vi "UHR-Fleezers Control (host) - Lorentz v2.vi"() -> ()   [LabVIEW 2014] (continued)
                  n2956 = local read "APD 2 Rate (Hz)"() -> (w4355:dbl)
                  n2957 = Multiply(x="Cy5 Fl.  Thresh. (kHz)", y=1000.0) -> (x*y=w4358:dbl)
                  n2958 = Greater?(x=w4355, y=w4358) -> (0:w4354:bool)
                  n2959 = And(x=w4354, y=w4351) -> (x .and. y?=w4352:bool)
                  n2960 = case shown="True" w4352 {
                    frame False {
                    }
                    frame True {
                      n2961 = property on="Green Laser ON" class="Bool (strict)"("Val(Sgnl)"=TRUE ("Value (Signaling)")) -> ()  [unwired: 2 in, 2 out]
                    }
                  }
                  n2962 = node-c288() -> ()  [unwired: 1 in, 1 out]
                }
                n2963 = node-c288(w4349) -> ()  [unwired: 1 out]
              }
              frame #4 {
                w4365 = FALSE ("Value (Signaling)")
                # "lower spot"
                n2964 = local read "Saved Stage Positions"() -> (w4369:dbl[][])
                n2965 = property on="Red Laser ON" class="Bool (strict)"("Val(Sgnl)"=w4365) -> ()  [unwired: 2 in, 2 out]
                n2966 = property on="Green Laser ON" class="Bool (strict)"("Val(Sgnl)"=w4365) -> ()  [unwired: 2 in, 2 out]
                n2967 = local write "Stage Moving"(TRUE ("Stage Moving")) -> ()
                n2968 = local write "Stop assembly line"(FALSE ("Stop assembly line")) -> ()
                n2969 = call "move to saved stage position.vi"("Stage VISA resource name in"=w4366, "Position"=3, "Saved Stage Positions"=w4369) -> ("error out"=w4368:errorcluster)  [unwired: 1 in, 1 out]
                n2970 = local write "Stage Control Serial Error"(w4368) -> ()
              }
              frame #5 {
                w4371 = FALSE ("Stage Moving")
                n2971 = local write "Stage Moving"(w4371) -> ()
                n2972 = local write "AL Running"(w4371) -> ()
                n2973 = call <vilib>:"Beep.vi"() -> ()  [unwired: 3 in, 9 out]
              }
            }
          }
        }
      }
      event "Stop All": Value Change {
        n2974 = event-data() -> ()  [unwired: 7 out]
        n2975 = local read "Stop All"() -> (w4372:bool)
      }
    }
    n2976 = node-c288() -> ()  [unwired: 2 out]
  }
  n2977 = node-c288(i64 1 ("Period"), 1 ("Processor")) -> (w68:T35)  [unwired: 2 in, 2 out]
  n2978 = node-c288(w29) -> ()  [unwired: 1 out]
  n2979 = node-c288(w61) -> ()  [unwired: 1 out]
  n2980 = node-c288(w63) -> ()  [unwired: 1 out]
  n2981 = node-c288(w51) -> ()  [unwired: 1 out]
  n2982 = property on="Saved trap pos" class="WFGraph (strict)"("Visible"=FALSE) -> ()  [unwired: 2 in, 2 out]
  n2983 = property on="Trap Delta Graph" class="WFGraph (strict)"("Visible"=TRUE) -> ()  [unwired: 2 in, 2 out]
  n2984 = disable-structure shown="Disabled" {
    disable-tunnel: w54 -> [w4374 _]
    disable-tunnel: w53 -> [w4373 _]
    frame Disabled {
      n2985 = VISA Close(VISA resource name=w4374, error in (no error)=w4373) -> (error out=w4375:errorcluster)
      n2986 = call <vilib>:"Simple Error Handler.vi"("error in (no error)"=w4375) -> ()  [unwired: 1 in, 8 out]
    }
    frame Enabled {
    }
  }
  n2987 = disable-structure shown="Disabled" {
    disable-tunnel: [w4383 _] -> w15
    disable-tunnel: [w4379 _] -> w14
    disable-tunnel: [w4378 _] -> w13
    disable-tunnel: [w4377 _] -> w12
    disable-tunnel: [w4376 _] -> w11
    frame Disabled {
      # "n samples needed for data"
      n2988 = Unbundle By Name("sound format") -> ("sample rate (S/s)"=w4379:dbl)
      n2989 = call <vilib>:"Sound Output Configure.vi"("number of samples/ch"="number of samples/ch", "sample mode"="sample mode", "sound format"="sound format", "device ID"="device ID") -> ("task ID"=w4383:T50)  [unwired: 6 in, 1 out]
      n2990 = local read "DMA Update Period (s)"() -> (w4380:dbl)
      n2991 = Multiply(x=w4380, y=w4379) -> (x*y=w4378:dbl)
      n2992 = for "Sound time base" {
        N: w4378 -> [_]
        tunnel: [w4387] -> w4381 mode=indexing
        i -> [w4387]
      }
      n2993 = Reciprocal(x=w4379) -> (1/x=w4377:dbl)
      n2994 = Multiply(x=w4381, y=w4377) -> (x*y=w4376:dbl[])
    }
    frame Enabled {
    }
  }
  n2995 = timed-loop "Main data acquisition loop (get data, process data for display, and save data to disk)" {
    tunnel: w10 -> [w4738]
    tunnel: w23 -> [w4737]
    tunnel: [w4765] -> w75
    tunnel: [w4760] -> w74
    timing: w68 -> [_]
    timing-out: [_] -> w67
    tunnel: w45 -> [w4627]
    tunnel: [w4459] -> w16
    tunnel: w15 -> [w4458]
    tunnel: w14 -> [w4456]
    tunnel: w13 -> [w4455]
    tunnel: w12 -> [w4454]
    tunnel: w11 -> [w4453]
    stop <- "Stop All" stop-if-true
    w4403 = 6.0  # clock mult.
    w4402 = 49152000.0  # TCXO frequ.
    w4544 = "Initialize"
    # "Added by Ronen - the limits imposed on amplitudes sent to AOM\nare not explicitly imposed when using intensity feedback. At amplitude of \n~48% FB intensity is ~1.8, if while feedback is on the value passes 1.8, feedback\nis turned off (indication that feedback algorithm overshoots)."
    # "Confocal image scanning disable by Ronen"
    # "List of channels in order (X or Y only):\nT1 X (mV)\nT2 X (mV)\nT1 X (nm)\nT2 X (nm)\nT1 FX (pN)\nT2 FX (pN)\nPosition Difference (nm)\nAPD1\nAPD2\nAPD3"
    # "T2 sum"
    # "T1 sum"
    # "Fluorescence data into FIFO for external control vi's\n(e.g., fluorescence triggering) - Duncan Nall"
    n2996 = node-c288() -> ()  [unwired: 2 out]
    n2997 = First Call?() -> (First Call?: T/F=w4579:bool)
    n2998 = Or(x="Reset", y=w4579) -> (x .or. y?=w4580:bool)
    n2999 = local read "Flushing P1"() -> (w4504:bool)
    n3000 = case "Reset data stream (manual reset or at begining of some rastering and imaging)" shown="True" w4580 {
      tunnel: w4738 -> [w5877 w5885]
      tunnel: w4737 -> [w5876 w5884]
      tunnel: [w5877 w5879] -> w4432
      tunnel: [w5876 w5878] -> w4433
      frame False {
      }
      frame True {
        w5882 = TRUE ("AI to FIFO")
        n3001 = local write "Overflow (data lost)"(FALSE ("Overflow (data lost)")) -> ()
        n3002 = call "reset FPGA DMA.vi"("error in"=w5884, "FPGA VI Reference In"=w5885) -> ("error out"=w5880:errorcluster, "FPGA VI Reference Out"=w5881:T31)
        n3003 = xnode "Read/Write Control"("FPGA VI Reference In"=w5881, "error in"=w5880, "AI to FIFO"=w5882, "APD to FIFO"=w5882) -> ("FPGA VI Reference Out"=w5879:T31, "error out"=w5878:errorcluster)
      }
    }
    n3004 = case shown="False" w4504 {
      frame False {
      }
      frame True {
        n3005 = local read "Flush rate (uL/m) P1"() -> (w4912:dbl)
        n3006 = local read "HP1 Flush Time (s)"() -> (w4921:dbl)
        n3007 = local read "DMA Update Period (s)"() -> (w4915:dbl)
        n3008 = Divide(x=w4912, y=60.0) -> (x/y=w4913:dbl)
        n3009 = Divide(x=w4921, y=w4915) -> (x/y=w4910:dbl)
        n3010 = feedback #4(0) -> (w4919:i32)
        n3011 = Increment(x=w4919) -> (x+1=w4909:i32)
        n3012 = Greater?(x=w4909, y=w4910) -> (0:w4918:bool)
        n3013 = Compound Arithmetic op=MULTIPLY(w4915, w4909, w4913) -> (→"P1 Flush Volume (uL)":dbl)
        n3014 = Divide(x=w4909, y=w4910) -> (x/y=→"P1 Flushing Bar":dbl)
        n3015 = case shown="True" w4918 {
          tunnel: w4909 -> [w4922 _]
          tunnel: [w4922 0] -> w4917
          frame False {
          }
          frame True {
            w4923 = FALSE ("Flushing P1")
            n3016 = local write "Inject Pump 1"(w4923) -> ()
            n3017 = local write "Flushing P1"(w4923) -> ()
            n3018 = property on="Clear Volume P1" class="Bool (strict)"("Val(Sgnl)"=TRUE ("Value (Signaling)")) -> ()  [unwired: 2 in, 2 out]
          }
        }
        n3019 = feedback-in #4(w4917) -> ()
      }
    }
    n3020 = Or(x="Start AOD Scan", y="Trap Raster Scan") -> (x .or. y?=w4700:bool)
    n3021 = case "Start active calibration (oscillate traps precisely)" shown="True" "Active Cal" {
      tunnel: w4433 -> [w4826 w4834]
      tunnel: w4432 -> [w4825 w4835]
      tunnel: [w4826 w4831] -> w4431
      tunnel: [w4825 w4832] -> w4430
      frame False {
      }
      frame True {
        w4827 = TRUE ("APD to FIFO")
        n3022 = call "reset FPGA DMA.vi"("error in"=w4834, "FPGA VI Reference In"=w4835) -> ("error out"=w4828:errorcluster, "FPGA VI Reference Out"=w4829:T31)
        n3023 = local write "Active Cal"(FALSE ("Active Cal")) -> ()
        n3024 = local write "Save Calibration"(TRUE ("Save Calibration")) -> ()
        n3025 = xnode "Read/Write Control"("FPGA VI Reference In"=w4829, "error in"=w4828, "AI to FIFO"=w4827, "APD to FIFO"=w4827) -> ("FPGA VI Reference Out"=w4832:T31, "error out"=w4831:errorcluster)
      }
    }
    n3026 = case "Start AOM raster scan" shown="True" w4700 {
      tunnel: w4430 -> [w5727 w5737]
      tunnel: w4431 -> [w5726 w5736]
      tunnel: [w5727 w5730] -> w4733
      tunnel: [w5726 w5729] -> w4732
      frame False {
      }
      frame True {
        n3027 = case shown="True" "Restart DMA? (AOD)" {
          tunnel: [w5775 w5777] -> w5731
          tunnel: [w5774 w5776] -> w5732
          tunnel: w5737 -> [w5775 w5779]
          tunnel: w5736 -> [w5774 w5778]
          frame False {
          }
          frame True {
            n3028 = local write "Overflow (data lost)"(FALSE ("Overflow (data lost)")) -> ()
            n3029 = call "reset FPGA DMA.vi"("error in"=w5778, "FPGA VI Reference In"=w5779) -> ("error out"=w5776:errorcluster, "FPGA VI Reference Out"=w5777:T31)
          }
        }
        n3030 = local write "Trap Raster Scan"(FALSE ("Trap Raster Scan")) -> ()
        n3031 = case shown="True" "Move MCL Also?" {
          tunnel: w5732 -> [w5740 w5769]
          tunnel: w5731 -> [w5741 w5770]
          tunnel: [w5739 w5773] -> w5730
          tunnel: [w5738 w5772] -> w5729
          frame False {
            w5742 = TRUE ("AI to FIFO")
            n3032 = xnode "Read/Write Control"("FPGA VI Reference In"=w5741, "error in"=w5740, "AI to FIFO"=w5742, "APD to FIFO"=w5742, "Start scan"=w5742) -> ("FPGA VI Reference Out"=w5739:T31, "error out"=w5738:errorcluster)
          }
          frame True {
            w5766 = FALSE ("1D or 2D Scan?")
            w5771 = TRUE ("AI to FIFO")
            # "Count for MCL loop"
            # "N total cycles"
            # "N steps"
            # "V_int"
            n3033 = local read "Scan Range (nm)"() -> (w5748:dbl)
            n3034 = local read "Number of F/B Scans (AOD)"() -> (w5765:u16)
            n3035 = Sign(1:w5748) -> (0:w5747:dbl)
            n3036 = Compound Arithmetic op=MULTIPLY(w5748, "MCL Step Position Ratio", "MCL/AOM Scale Tweak") -> (w5752:dbl)
            n3037 = Negate(x=w5747) -> (-x=w5744:dbl)
            n3038 = Multiply(x=w5744, y="MCL Step Increment (V_int)") -> (x*y=w5746:dbl)
            n3039 = Divide(x=w5752, y="MCL X Cal (nm/V)") -> (x/y=w5758:dbl)
            n3040 = Multiply(x=32767.0 ("y"), y=w5758) -> (x*y=w5764:dbl)
            n3041 = local read "Total Counts (ticks)"() -> (w5749:u16)
            n3042 = local read "Cycles/step (AOD)"() -> (w5760:u64)
            n3043 = local read "Scan steps (AOD)"() -> (w5761:u64)
            n3044 = Divide(x=w5764, y=10.0) -> (x/y=w5757:dbl)
            n3045 = Divide(x=w5757, y="MCL Step Increment (V_int)") -> (x/y=w5755:dbl)
            n3046 = Absolute Value(x=w5755) -> (abs(x)=w5743:dbl)
            n3047 = Compound Arithmetic op=MULTIPLY(w5761, w5760, w5749) -> (w5756:u64)
            n3048 = Divide(x=w5756, y=w5743) -> (x/y=w5753:dbl)
            "MCL Count" <- w5753
            n3049 = xnode "Read/Write Control"("FPGA VI Reference In"=w5770, "error in"=w5769, "Scan steps (MCL)"=w5743, "Number of scans (MCL)"=w5765, "Cycles per step (MCL)"=u64 1, "Scan freq.  increment (MCL)"=w5746, "1D or 2D Scan?"=w5766, "MCL Scan Axis"=w5766, "Cont. Scan (MCL)"=w5766, "MCL count"=w5753) -> ("FPGA VI Reference Out"=w5768:T31, "error out"=w5767:errorcluster)
            n3050 = xnode "Read/Write Control"("FPGA VI Reference In"=w5768, "error in"=w5767, "AI to FIFO"=w5771, "APD to FIFO"=w5771, "Start scan"=w5771, "Start scan (MCL)"=w5771) -> ("FPGA VI Reference Out"=w5773:T31, "error out"=w5772:errorcluster)
            n3051 = local write "MCL Scanning"(w5771) -> ()
            n3052 = local write "wait to reset values"(w5771) -> ()
          }
        }
        "Raster Scanning..." <- TRUE ("Scanning...")
      }
    }
    n3053 = local read "Flushing P3"() -> (w4505:bool)
    n3054 = case "Keep track of when Harvard Pump 3 is done flushing" shown="True" w4505 {
      frame False {
      }
      frame True {
        n3055 = local read "Flush rate (uL/m) P3"() -> (w4929:dbl)
        n3056 = local read "DMA Update Period (s)"() -> (w4931:dbl)
        n3057 = local read "HP3 Flush Time (s)"() -> (w4938:dbl)
        n3058 = Divide(x=w4929, y=60.0) -> (x/y=w4927:dbl)
        n3059 = feedback #5(0) -> (w4936:i32)
        n3060 = Increment(x=w4936) -> (x+1=w4930:i32)
        n3061 = Divide(x=w4938, y=w4931) -> (x/y=w4932:dbl)
        n3062 = Greater?(x=w4930, y=w4932) -> (0:w4935:bool)
        n3063 = Compound Arithmetic op=MULTIPLY(w4931, w4930, w4927) -> (→"P3 Flush Volume (uL)":dbl)
        n3064 = case shown="True" w4935 {
          tunnel: w4930 -> [w4939 _]
          tunnel: [w4939 0] -> w4934
          frame False {
          }
          frame True {
            w4940 = FALSE ("Flushing P3")
            n3065 = local write "Inject Pump 3"(w4940) -> ()
            n3066 = local write "Flushing P3"(w4940) -> ()
            n3067 = property on="Clear Volume P3" class="Bool (strict)"("Val(Sgnl)"=TRUE ("Value (Signaling)")) -> ()  [unwired: 2 in, 2 out]
          }
        }
        n3068 = feedback-in #5(w4934) -> ()
        n3069 = Divide(x=w4930, y=w4932) -> (x/y=→"P3 Flushing Bar":dbl)
      }
    }
    n3070 = And(x="Save scans", y=w4700) -> (x .and. y?=w4731:bool)
    n3071 = Compound Arithmetic op=OR("Start MCL Scan", "Confocal Image", "Confocal Linescan") -> (w4698:bool)
    n3072 = And(x="Save Data (MCL)", y=w4698) -> (x .and. y?=w4730:bool)
    n3073 = case "Start MCL raster scan" shown="True" w4698 {
      tunnel: w4733 -> [w5339 w5355]
      tunnel: w4732 -> [w5338 w5354]
      tunnel: [w5339 w5350] -> w4626
      tunnel: [w5338 w5349] -> w4625
      tunnel: [FALSE w5348] -> w4716
      tunnel: "Start MCL Scan" -> [_ w5343]
      tunnel: "Confocal Image" -> [_ w5342]
      tunnel: "Confocal Linescan" -> [_ _]
      frame False {
      }
      frame True {
        w5348 = TRUE
        n3074 = case shown="True" "Restart DMA? (MCL)" {
          tunnel: [w5400 w5402] -> w5353
          tunnel: [w5399 w5401] -> w5352
          tunnel: w5355 -> [w5400 w5405]
          tunnel: w5354 -> [w5399 w5404]
          frame False {
          }
          frame True {
            n3075 = call "reset FPGA DMA.vi"("error in"=w5404, "FPGA VI Reference In"=w5405) -> ("error out"=w5401:errorcluster, "FPGA VI Reference Out"=w5402:T31)
            n3076 = local write "Overflow (data lost)"(FALSE ("Overflow (data lost)")) -> ()
          }
        }
        n3077 = case shown="False" w5343 {
          selector: w5343 -> [_ w5359]
          tunnel: w5342 -> [w5358 _]
          tunnel: [w5358 w5359] -> w5341
          frame False {
            n3078 = property on="2D or 1D Scan" class="Bool (strict)"("Val(Sgnl)"=w5358) -> ()  [unwired: 2 in, 2 out]
            n3079 = property on="Confocal Image" class="Bool (strict)"("Value"=FALSE ("Start Confocal Map")) -> ()  [unwired: 2 in, 2 out]
          }
          frame True {
          }
        }
        n3080 = local write "MCL Scanning"(w5348) -> ()
        n3081 = local read "AO1"() -> (w5345:dbl)
        n3082 = local read "AO2"() -> (w5344:dbl)
        n3083 = case shown="True" "Center Scan" {
          tunnel: w5353 -> [w5366 w5398]
          tunnel: w5352 -> [w5365 w5397]
          tunnel: [w5364 w5396] -> w5350
          tunnel: [w5363 w5395] -> w5349
          tunnel: [w5361 w5382] -> w5347
          tunnel: [w5360 w5381] -> w5346
          tunnel: w5345 -> [w5361 w5387]
          tunnel: w5344 -> [w5360 w5390]
          tunnel: w5341 -> [_ _]
          frame False {
            w5362 = TRUE ("AI to FIFO")
            n3084 = xnode "Read/Write Control"("FPGA VI Reference In"=w5366, "error in"=w5365, "AI to FIFO"=w5362, "APD to FIFO"=w5362, "Start scan (MCL)"=w5362) -> ("FPGA VI Reference Out"=w5364:T31, "error out"=w5363:errorcluster)
          }
          frame True {
            w5394 = TRUE ("AI to FIFO")
            n3085 = local read "Scan steps (MCL)"() -> (w5373:u64)
            n3086 = local read "Scan lines (y)"() -> (w5369:u64)
            n3087 = local read "Fast Scan Dir"() -> (w5380:bool)
            n3088 = local read "Actual MCL Inc (V)"() -> (w5370:dbl)
            n3089 = Decrement(x=w5369) -> (x-1=w5368:u64)
            n3090 = Decrement(x=w5373) -> (x-1=w5372:u64)
            n3091 = Multiply(x=w5370, y=w5368) -> (x*y=w5367:dbl)
            n3092 = Divide(x=w5367, y=2.0) -> (x/y=w5377:dbl)
            n3093 = Multiply(x=w5370, y=w5372) -> (x*y=w5371:dbl)
            n3094 = Divide(x=w5371, y=2.0) -> (x/y=w5376:dbl)
            n3095 = Select(t=w5376, s=w5380, f=w5377) -> (s? t:f=w5375:dbl)
            n3096 = Select(t=w5377, s=w5380, f=w5376) -> (s? t:f=w5379:dbl)
            n3097 = Subtract(x=w5387, y=w5379) -> (x-y=w5378:dbl)
            n3098 = Subtract(x=w5390, y=w5375) -> (x-y=w5374:dbl)
            n3099 = local read "2D or 1D Scan"() -> (w5392:bool)
            n3100 = Not(x=w5380) -> (.not. x?=w5386:bool)
            n3101 = Not(x=w5392) -> (.not. x?=w5388:bool)
            n3102 = And(x=w5380, y=w5388) -> (x .and. y?=w5389:bool)
            n3103 = And(x=w5388, y=w5386) -> (x .and. y?=w5391:bool)
            n3104 = Select(t=w5390, s=w5391, f=w5374) -> (s? t:f=w5381:dbl)
            n3105 = Select(t=w5387, s=w5389, f=w5378) -> (s? t:f=w5382:dbl)
            n3106 = call "Volt to I16.vi"("Voltage In"=w5382) -> ("I16 Voltage Out"=w5385:i16)
            n3107 = call "Volt to I16.vi"("Voltage In"=w5381) -> ("I16 Voltage Out"=w5384:i16)
            n3108 = xnode "Read/Write Control"("FPGA VI Reference In"=w5398, "error in"=w5397, "AI to FIFO"=w5394, "APD to FIFO"=w5394, "Start scan (MCL)"=w5394, "AO1"=w5385, "AO2"=w5384) -> ("FPGA VI Reference Out"=w5396:T31, "error out"=w5395:errorcluster)
          }
        }
        "Initial Y" <- w5347
        "Initial X" <- w5346
        n3109 = local write "Tab Control 6"(T3."Imaging" ("Tab Control 6")) -> ()
        "wait to reset values" <- w5348
      }
    }
    n3110 = local read "APD Elements/DMA read"() -> (w4475:u32)
    n3111 = local read "Trap AI Elements/DMA read"() -> (w4679:u32)
    n3112 = xnode "Get APD Data"("FPGA VI Reference In"=w4626, "error in"=w4625, "Number of Elements"=w4475, "Timeout (ms)"=-1) -> ("Data"=w4654:void[], "Elements Remaining"=→"APD FIFO Elements Remaining")  [unwired: 2 out]
    n3113 = local read "Trap Pos Elements/DMA read"() -> (w4622:u32)
    n3114 = xnode "Invoke Method"("FPGA VI Reference In"=w4626, "error in"=w4625, "Number of Elements"=w4622, "Timeout (ms)"=-1) -> ("Data"=w4586:void[], "Elements Remaining"=→"Trap Pos FIFO El Remaining")  [unwired: 2 out]
    n3115 = xnode "Get Trap Data"("FPGA VI Reference In"=w4626, "error in"=w4625, "Number of Elements"=w4679, "Timeout (ms)"=-1 ("Timeout")) -> ("FPGA VI Reference Out"=w4401:T31, "error out"=w4522:errorcluster, "Data"=w4587:void[], "Elements Remaining"=w4773)
    "FIFO El. Rem." <- w4773
    n3116 = local read "DMA Update Period (s)"() -> (w4680:dbl)
    n3117 = local read "Trap AI FIFO Depth"() -> (w4775:u32)
    n3118 = local read "Number of APDs"() -> (w4494:u8)
    n3119 = Decimate 1D Array(w4586) -> (w4583:void[], w4585:void[], w4584:void[])
    n3120 = feedback #6(0.0) -> (w4615:dbl)
    n3121 = Add(x=w4680, y=w4615) -> (x+y=w4750:dbl)
    n3122 = feedback-in #6(w4750) -> ()
    n3123 = To Time Stamp(1:w4615) -> (0:w4614:timestamp)
    n3124 = Subtract(x=w4775, y=w4679) -> (x-y=w4774:u32)
    n3125 = To Unsigned Long Integer(number=w4583) -> (unsigned 32bit integer=w4582:u32[])
    n3126 = Join Numbers(hi=w4585, lo=w4584) -> ((hi.lo)=w4581:u32)
    n3127 = Divide(x=w4773, y=w4774) -> (x/y=w4772:dbl)
    "Buffer Status" <- w4772
    n3128 = case "Deinterlace APD signals" shown="3, Default" w4494 {
      tunnel: [w4902 w4908] -> w4474
      tunnel: w4654 -> [w4903 w4907]
      tunnel: [w4901 w4906] -> w4473
      tunnel: [w4900 w4904] -> w4422
      frame 3, Default {
        n3129 = Decimate 1D Array "APD signals"(w4903) -> (w4902:void[], w4901:void[], w4900:void[])
      }
      frame 2 {
        n3130 = Decimate 1D Array "APD signals"(w4907) -> (w4908:void[], w4906:void[])
        n3131 = Multiply(x=w4906, y=u32 0) -> (x*y=w4904:u32)
      }
    }
    n3132 = Join Numbers(hi=w4582, lo=w4581) -> ((hi.lo)=w4575:u64[])
    n3133 = call "IR AOM word to freq - vec.vi"("Frequency Word In (double vec)"=w4575) -> ("Frequency Out"=w4621:dbl[])
    n3134 = Equal?(x=w4772, y=1.0) -> (x = y?=w4770:bool)
    n3135 = case "Alert buffer overflow" shown="False" w4770 {
      frame False {
      }
      frame True {
        n3136 = call <vilib>:"Beep.vi"() -> ()  [unwired: 3 in, 9 out]
        "Overflow (data lost)" <- TRUE ("Overflow (data lost)")
      }
    }
    n3137 = Decimate 1D Array(w4621) -> (w4620:dbl[], w4619:dbl[])
    n3138 = Build Array(w4620, w4619) -> (w4618:dbl[][])
    n3139 = Bundle(w4474, w4473, w4422) -> (w4478:cluster{void[], void[], u32})  [unwired: 1 in]
    n3140 = Build Array(w4474, w4473, w4422) -> (w4713:u32[])
    n3141 = for {
      tunnel: w4474 -> [w4898] mode=indexing
      n3142 = call "Smart Buffer (DBL) 1.vi"("new element [write]"=w4898, "mode"=T33."write") -> ()  [unwired: 4 in, 6 out]
    }
    n3143 = local read "APD Integration Time (s)"() -> (w4489:dbl)
    n3144 = To Double Precision Float(number=w4713) -> (double precision float=w4714:dbl[])
    n3145 = feedback #7 "APD3"(w4422) -> (w4423:u32)
    n3146 = feedback #8 "APD2"(w4473) -> (w4644:void[])
    n3147 = feedback #9 "APD1"(w4474) -> (w4712:void[])
    n3148 = Build Array(w4423, w4422) -> (w4421:u32[])
    n3149 = Build Array (concatenate)(w4644, w4473) -> (w4643:void[])
    n3150 = Build Array (concatenate)(w4712, w4474) -> (w4709:void[])
    n3151 = for {
      tunnel: w4473 -> [w4897] mode=indexing
      n3152 = call "Smart Buffer (DBL) 2.vi"("new element [write]"=w4897, "mode"=T33."write") -> ()  [unwired: 4 in, 6 out]
    }
    n3153 = Array Size(array=w4709) -> (size(s)=w4706:i32)
    n3154 = Array Size(array=w4474) -> (size(s)=w4708:i32)
    n3155 = Multiply(x=w4708, y="APD Ave N") -> (x*y=w4707:dbl)
    n3156 = Greater?(x=w4706, y=w4707) -> (0:w4710:bool)
    n3157 = Bundle("APD 1", "APD 2", "APD 3") -> (w4744:cluster{string, string, string})  [unwired: 1 out]
    n3158 = local read "Trap Sets"() -> (w4678:u32)
    n3159 = case shown="True" w4710 {
      tunnel: w4709 -> [w5154 w5163]
      tunnel: [w5154 w5161] -> w4685
      tunnel: w4707 -> [_ w5156]
      tunnel: w4706 -> [_ w5162]
      tunnel: w4643 -> [w5153 w5160]
      tunnel: [w5153 w5159] -> w4641
      tunnel: w4421 -> [w5152 w5158]
      tunnel: [w5152 w5155] -> w4490
      frame False {
      }
      frame True {
        n3160 = Subtract(x=w5162, y=w5156) -> (x-y=w5157:dbl)
        n3161 = Array Subset "APD3"(array=w5158, index=w5157, length=w5156) -> (w5155:u32[])
        n3162 = Array Subset "APD2"(array=w5160, index=w5157, length=w5156) -> (w5159:void[])
        n3163 = Array Subset "APD1"(array=w5163, index=w5157, length=w5156) -> (w5161:void[])
      }
    }
    n3164 = feedback-in #7(w4490) -> ()
    n3165 = feedback-in #8(w4641) -> ()
    n3166 = feedback-in #9(w4685) -> ()
    n3167 = Cluster To Array(cluster=w4744) -> (array=w4741:string[])
    n3168 = for "APD" {
      tunnel: w4714 -> [w5410] mode=indexing
      tunnel: w4489 -> [w5417]
      tunnel: [w5413] -> w4645 mode=indexing
      tunnel: "APD Disp. Scale" -> [w5414]
      tunnel: w4741 -> [w5412] mode=indexing
      tunnel: "APD Disp. Downsample" -> [w5408]
      tunnel: [w5411] -> w4740
      workers-P: _ -> [_]
      tunnel: w4614 -> [w5407]
      n3169 = call "integrate 1D array interval - double.vi"("Ave N"=w5408, "Array In"=w5410) -> ("Array Out"=w5409:dbl[])  [unwired: 1 out]
      n3170 = Multiply(x=w5417, y=w5408) -> (x*y=w5411:dbl)
      n3171 = Divide(x=w5409, y=w5414) -> (x/y=w5415:dbl[])
      n3172 = Bundle By Name("t0"=w5407, "Y"=w5415, "dt"=w5411) -> (w5416:waveform(dbl))  [unwired: 1 out]
      n3173 = Set Waveform Attribute(5:w5412, 6:"NI_ChannelName" ("name"), 7:w5416) -> (3:w5413:waveform(dbl))  [unwired: 1 in, 2 out]
    }
    "APD Display Period (s)" <- w4740
    n3174 = Reciprocal(x=w4740) -> (1/x=→"APD Display Freq. (Hz)":dbl)
    n3175 = case "Deinterlace trap data, average down PSD" shown="2" w4678 {
      tunnel: w4587 -> [w5435 w5500]
      tunnel: [w5432 w5497] -> w4673
      tunnel: [w5435 w5499] -> w4578
      tunnel: "Detector Type" -> [w5434 w5495]
      tunnel: [w5433 w5498] -> w4672
      tunnel: [w5431 w5496] -> w4748
      frame 1, Default {
        n3176 = Divide(x=w5435, y=3276.7) -> (x/y=w5436:dbl)
        n3177 = Decimate 1D Array(w5436) -> (w5445:dbl[], w5444:dbl[], w5443:dbl[], w5442:dbl[], w5441:dbl[], w5440:dbl[], w5439:dbl[], w5438:dbl[])
        n3178 = case shown="\"IR-QPD + PSD + FB-QPD position\"" w5434 {
          tunnel: w5445 -> [w5469 w5494]
          tunnel: w5444 -> [w5468 w5493]
          tunnel: w5443 -> [w5453 w5471]
          tunnel: w5442 -> [w5454 w5481]
          tunnel: w5441 -> [w5467 w5492]
          tunnel: w5440 -> [w5466 w5491]
          tunnel: w5439 -> [w5450 w5472]
          tunnel: w5438 -> [w5449 w5470]
          tunnel: [w5448 w5478] -> w5433
          tunnel: [w5447 w5477] -> w5432
          tunnel: [w5446 w5476] -> w5431
          frame "IR-QPD + PSD + FB-QPD", Default {
            w5446 = 0  # Channel pattern
            n3179 = Divide(x=w5469, y=w5454) -> (x/y=w5456:dbl[])
            n3180 = Divide(x=w5468, y=w5454) -> (x/y=w5455:dbl[])
            n3181 = Divide(x=w5467, y=w5450) -> (x/y=w5452:dbl[])
            n3182 = Divide(x=w5466, y=w5449) -> (x/y=w5451:dbl[])
            n3183 = Build Array(w5456, w5455, w5454, w5453, w5452, w5451, w5450, w5449) -> (w5447:dbl[][])
            n3184 = Bundle("T1 Y", "T1 X", "T1 Sum", "FB Sum", "PSD Y", "PSD X", "PSD Y Sum", "PSD X Sum") -> (w5465:T57)  [unwired: 1 out]
            n3185 = Cluster To Array(cluster=w5465) -> (array=w5448:string[])
          }
          frame "IR-QPD + PSD + FB-QPD position" {
            w5476 = 3  # Channel pattern
            n3186 = Negate(x=w5472) -> (-x=w5473:dbl[])
            n3187 = Divide(x=w5494, y=w5481) -> (x/y=w5483:dbl[])
            n3188 = Divide(x=w5493, y=w5481) -> (x/y=w5482:dbl[])
            n3189 = Divide(x=w5492, y=w5472) -> (x/y=w5480:dbl[])
            n3190 = Divide(x=w5491, y=w5473) -> (x/y=w5479:dbl[])
            n3191 = Build Array(w5483, w5482, w5481, w5470, w5471, w5480, w5479, w5472) -> (w5477:dbl[][])
            n3192 = Bundle("T1 Y", "T1 X", "T1 Sum", "FB X", "FB Sum", "PSD Y", "PSD X", "PSD Y Sum") -> (w5490:T57)  [unwired: 1 out]
            n3193 = Cluster To Array(cluster=w5490) -> (array=w5478:string[])
          }
        }
      }
      frame 2 {
        n3194 = case shown="\"IR-QPD + PSD + FB-QPD X position\", Default" w5495 {
          tunnel: w5500 -> [w5562 w5634 w5705]
          tunnel: [w5501 w5625 w5636] -> w5499
          tunnel: [w5528 w5616 w5683] -> w5498
          tunnel: [w5527 w5579 w5650] -> w5497
          tunnel: [w5521 w5614 w5681] -> w5496
          frame "IR-QPD + PSD + FB-QPD" {
            w5521 = 1  # Channel pattern
            # "time average x2 the 4th signal and the 4 psd signals (detection laser)"
            # "deinterlace 3 signals from qpd"
            n3195 = Decimate 1D Array(w5562) -> (w5561:void[], w5560:void[], w5526:void[], w5559:void[], w5549:void[], w5547:void[], w5546:void[], w5544:void[])
            n3196 = Decimate 1D Array(w5526) -> (w5525:void[], w5524:void[])
            n3197 = Decimate 1D Array(w5561) -> (w5558:void[], w5530:void[])
            n3198 = Decimate 1D Array(w5560) -> (w5557:void[], w5555:void[])
            n3199 = Decimate 1D Array(w5559) -> (w5556:void[], w5554:void[])
            n3200 = call "downsample 1D array - double.vi"("Ave N"=2.0, "Array In"=w5549) -> ("Array Out"=w5548:dbl[])  [unwired: 1 out]
            n3201 = call "downsample 1D array - double.vi"("Ave N"=2.0, "Array In"=w5547) -> ("Array Out"=w5529:dbl[])  [unwired: 1 out]
            n3202 = call "downsample 1D array - double.vi"("Ave N"=2.0, "Array In"=w5546) -> ("Array Out"=w5545:dbl[])  [unwired: 1 out]
            n3203 = call "downsample 1D array - double.vi"("Ave N"=2.0, "Array In"=w5544) -> ("Array Out"=w5543:dbl[])  [unwired: 1 out]
            n3204 = Interleave 1D Arrays(w5558, w5557, w5556, w5530, w5555, w5554, w5525, w5524, w5548, w5529, w5545, w5543) -> (w5542:dbl[])
            n3205 = Divide(x=w5542, y=3276.7) -> (x/y=w5541:dbl[])
            n3206 = Decimate 1D Array(w5541) -> (w5540:dbl[], w5539:dbl[], w5538:dbl[], w5537:dbl[], w5536:dbl[], w5535:dbl[], w5523:dbl[], w5522:dbl[], w5534:dbl[], w5533:dbl[], w5532:dbl[], w5531:dbl[])
            n3207 = Divide(x=w5540, y=w5538) -> (x/y=w5508:dbl[])
            n3208 = Divide(x=w5539, y=w5538) -> (x/y=w5507:dbl[])
            n3209 = Divide(x=w5537, y=w5535) -> (x/y=w5506:dbl[])
            n3210 = Divide(x=w5536, y=w5535) -> (x/y=w5505:dbl[])
            n3211 = Divide(x=w5534, y=w5532) -> (x/y=w5504:dbl[])
            n3212 = Divide(x=w5533, y=w5531) -> (x/y=w5503:dbl[])
            n3213 = Build Array(w5508, w5507, w5538, w5506, w5505, w5535, w5523, w5522, w5504, w5503, w5532, w5531) -> (w5527:dbl[][])
            n3214 = Bundle("T1 Y", "T1 X", "T1 Sum", "T2 Y", "T2 X", "T2 Sum", "T1 FB Sum", "T2 FB Sum", "PSD Y", "PSD X", "PSD Y Sum", "PSD X Sum") -> (w5509:T58)  [unwired: 1 out]
            n3215 = To Word Integer(number=w5542) -> (16bit integer=w5501:i16[])
            n3216 = Cluster To Array(cluster=w5509) -> (array=w5528:string[])
          }
          frame "IR-QPD + PSD + FB-QPD X position", Default {
            w5614 = 2  # Channel pattern
            # "time average x2 the 3 psd signals (detection laser)"
            # "deinterlace 3 signals from qpds"
            n3217 = Decimate 1D Array(w5634) -> (w5633:void[], w5632:void[], w5615:void[], w5631:void[], w5577:void[], w5574:void[], w5571:void[], w5602:void[])
            n3218 = Select(t=i16 -1, s="Flip X Sign", f=i16 1) -> (s? t:f=w5567:i16)
            n3219 = Multiply(x=w5632, y=w5567) -> (x*y=w5568:i16)
            n3220 = Decimate 1D Array(w5615) -> (w5600:void[], w5598:void[])
            n3221 = Decimate 1D Array(w5633) -> (w5630:void[], w5617:void[])
            n3222 = Decimate 1D Array(w5568) -> (w5629:dbl[], w5627:dbl[])
            n3223 = Decimate 1D Array(w5631) -> (w5628:void[], w5626:void[])
            n3224 = Decimate 1D Array(w5602) -> (w5601:void[], w5599:void[])
            n3225 = call "downsample 1D array - I16.vi"("Ave N"=2.0, "Array In"=w5577) -> ("Array Out"=w5575:i16[])  [unwired: 1 in]
            n3226 = call "downsample 1D array - I16.vi"("Ave N"=2.0, "Array In"=w5571) -> ("Array Out"=w5569:i16[])  [unwired: 1 in]
            n3227 = call "downsample 1D array - I16.vi"("Ave N"=2.0, "Array In"=w5574) -> ("Array Out"=w5572:i16[])  [unwired: 1 in]
            n3228 = Interleave 1D Arrays(w5630, w5629, w5628, w5617, w5627, w5626, w5601, w5600, w5599, w5598, w5575, w5572, w5569) -> (w5625:dbl[])
            n3229 = Divide(x=w5625, y=3276.7) -> (x/y=w5624:dbl[])
            n3230 = Decimate 1D Array(w5624) -> (w5623:dbl[], w5622:dbl[], w5621:dbl[], w5620:dbl[], w5619:dbl[], w5618:dbl[], w5590:dbl[], w5588:dbl[], w5587:dbl[], w5585:dbl[], w5584:dbl[], w5583:dbl[], w5580:dbl[])
            n3231 = Negate(x=w5580) -> (-x=w5578:dbl[])
            n3232 = Divide(x=w5584, y=w5580) -> (x/y=w5582:dbl[])
            n3233 = Divide(x=w5583, y=w5578) -> (x/y=w5581:dbl[])
            n3234 = Divide(x=w5623, y=w5621) -> (x/y=w5606:dbl[])
            n3235 = Divide(x=w5622, y=w5621) -> (x/y=w5605:dbl[])
            n3236 = Divide(x=w5620, y=w5618) -> (x/y=w5604:dbl[])
            n3237 = Divide(x=w5619, y=w5618) -> (x/y=w5603:dbl[])
            n3238 = Divide(x=w5590, y=w5588) -> (x/y=w5589:dbl[])
            n3239 = Divide(x=w5587, y=w5585) -> (x/y=w5586:dbl[])
            n3240 = Build Array(w5606, w5605, w5621, w5604, w5603, w5618, w5589, w5588, w5586, w5585, w5582, w5581, w5580) -> (w5579:dbl[][])
            n3241 = Bundle("T1 Y", "T1 X", "T1 Sum", "T2 Y", "T2 X", "T2 Sum", "T1 FB X", "T1 FB Sum", "T2 FB X", "T2 FB Sum", "PSD Y", "PSD X", "PSD Y Sum") -> (w5607:T59)  [unwired: 1 out]
            n3242 = Cluster To Array(cluster=w5607) -> (array=w5616:string[])
          }
          frame "IR-QPD + PSD + FB-QPD XY positions" {
            w5681 = 4  # Channel pattern
            # "time average x2 the 3 psd signals (detection laser)"
            # "deinterlace 3 signals from qpds"
            n3243 = Decimate 1D Array(w5705) -> (w5704:void[], w5703:void[], w5682:void[], w5702:void[], w5648:void[], w5694:void[], w5693:void[], w5670:void[])
            n3244 = Decimate 1D Array "Feedback Sum"(w5682) -> (w5666:void[], w5664:void[])
            n3245 = Decimate 1D Array "QPD Y"(w5704) -> (w5701:void[], w5684:void[])
            n3246 = Decimate 1D Array "QPD X"(w5703) -> (w5700:void[], w5698:void[])
            n3247 = Decimate 1D Array "Feedback Y"(w5648) -> (w5647:void[], w5646:void[])
            n3248 = Decimate 1D Array "QPD Sum"(w5702) -> (w5699:void[], w5697:void[])
            n3249 = Decimate 1D Array "Feedback X"(w5670) -> (w5667:void[], w5665:void[])
            n3250 = call "downsample 1D array - double.vi"("Ave N"=2.0, "Array In"=w5694) -> ("Array Out"=w5669:dbl[])  [unwired: 1 out]
            n3251 = call "downsample 1D array - double.vi"("Ave N"=2.0, "Array In"=w5693) -> ("Array Out"=w5668:dbl[])  [unwired: 1 out]
            n3252 = Interleave 1D Arrays(w5701, w5700, w5699, w5684, w5698, w5697, w5647, w5667, w5666, w5646, w5665, w5664, w5669, w5668) -> (w5692:dbl[])
            n3253 = Divide(x=w5692, y=3276.7) -> (x/y=w5691:dbl[])
            n3254 = Decimate 1D Array(w5691) -> (w5690:dbl[], w5689:dbl[], w5688:dbl[], w5687:dbl[], w5686:dbl[], w5685:dbl[], w5643:dbl[], w5657:dbl[], w5641:dbl[], w5642:dbl[], w5655:dbl[], w5639:dbl[], w5653:dbl[], w5651:dbl[])
            n3255 = Negate(x=w5651) -> (-x=w5649:dbl[])
            n3256 = Divide(x=w5653, y=w5649) -> (x/y=w5652:dbl[])
            n3257 = Divide(x=w5642, y=w5639) -> (x/y=w5638:dbl[])
            n3258 = Divide(x=w5643, y=w5641) -> (x/y=w5640:dbl[])
            n3259 = Divide(x=w5690, y=w5688) -> (x/y=w5674:dbl[])
            n3260 = Divide(x=w5689, y=w5688) -> (x/y=w5673:dbl[])
            n3261 = Divide(x=w5687, y=w5685) -> (x/y=w5672:dbl[])
            n3262 = Divide(x=w5686, y=w5685) -> (x/y=w5671:dbl[])
            n3263 = Divide(x=w5657, y=w5641) -> (x/y=w5656:dbl[])
            n3264 = Divide(x=w5655, y=w5639) -> (x/y=w5654:dbl[])
            n3265 = Build Array(w5674, w5673, w5688, w5672, w5671, w5685, w5640, w5656, w5641, w5638, w5654, w5639, w5652, w5651) -> (w5650:dbl[][])
            n3266 = Bundle("T1 Y", "T1 X", "T1 Sum", "T2 Y", "T2 X", "T2 Sum", "T1 FB Y", "T1 FB X", "T1 FB Sum", "T2 FB Y", "T2 FB X", "T2 FB Sum", "PSD X", "PSD Y Sum") -> (w5637:T60)  [unwired: 1 out]
            n3267 = To Word Integer(number=w5692) -> (16bit integer=w5636:i16[])
            n3268 = Cluster To Array(cluster=w5637) -> (array=w5683:string[])
          }
        }
      }
    }
    "AI labels" <- w4672
    n3269 = local read "APD Integration Time (s)"() -> (w4650:dbl)
    n3270 = Array Size(array=w4685) -> (size(s)=w4705:i32)
    n3271 = call <vilib>:"Std Deviation and Variance.vi"("X"=w4641) -> ("standard deviation"=w4640:dbl)  [unwired: 1 in, 2 out]
    n3272 = Add Array Elements(numeric array=w4641) -> (sum=w4642:dbl)
    n3273 = Add Array Elements(numeric array=w4685) -> (sum=w4715:dbl)
    n3274 = call <vilib>:"Std Deviation and Variance.vi"("X"=w4685) -> ("standard deviation"=w4684:dbl)  [unwired: 1 in, 2 out]
    n3275 = Divide(x=w4640, y=w4489) -> (x/y=w4637:dbl)
    "Rate sigma (Hz) 2" <- w4637
    n3276 = Multiply(x=w4489, y=w4705) -> (x*y=w4491:dbl)
    "Int. Time (s)" <- w4491
    n3277 = Divide(x=w4642, y=w4491) -> (x/y=w4638:dbl)
    "APD 2 Rate (Hz)" <- w4638
    n3278 = Multiply(x="APD Disp. Scale", y=w4645) -> (x*y=w4652:waveform(dbl)[])
    n3279 = Divide(x=w4715, y=w4491) -> (x/y=w4682:dbl)
    "APD 1 Rate (Hz)" <- w4682
    n3280 = Divide(x=w4684, y=w4489) -> (x/y=w4683:dbl)
    "Rate sigma (Hz)" <- w4683
    n3281 = Divide(x=w4637, y=w4638) -> (x/y=→"Sigma/Mean 2":dbl)
    n3282 = Multiply(x="APD Disp. Downsample", y=w4650) -> (x*y=w4648:dbl)
    n3283 = Divide(x=w4683, y=w4682) -> (x/y=→"Sigma/Mean":dbl)
    n3284 = Divide(x=w4652, y=w4648) -> (x/y=w4481:waveform(dbl)[])
    n3285 = Index Array(array=w4481, index=0) -> (element=w4634:waveform(dbl))
    n3286 = Index Array(array=w4481, index=1) -> (element=w4632:waveform(dbl))
    n3287 = Index Array(array=w4481, index=2) -> (element=w4483:waveform(dbl))
    n3288 = Subtract(x=w4634, y="APD 1 Offset") -> (x-y=w4630:waveform(dbl))
    n3289 = Subtract(x=w4632, y="APD 2 Offset") -> (x-y=w4629:waveform(dbl))
    n3290 = Subtract(x=w4483, y="APD 3 Offset") -> (x-y=w4480:waveform(dbl))
    n3291 = Add Array Elements(numeric array=w4490) -> (sum=w4493:u32)
    n3292 = call <vilib>:"Std Deviation and Variance.vi"("X"=w4490) -> ("standard deviation"=w4492:dbl)  [unwired: 1 in, 2 out]
    n3293 = Build Array(w4630, w4629, w4480) -> (→"APD Chart":waveform(dbl)[])
    n3294 = Divide(x=w4493, y=w4491) -> (x/y=w4487:dbl)
    "APD 3 Rate (Hz)" <- w4487
    n3295 = Divide(x=w4492, y=w4489) -> (x/y=w4488:dbl)
    "Rate sigma (Hz) 3" <- w4488
    n3296 = Divide(x=w4488, y=w4487) -> (x/y=→"Sigma/Mean 3":dbl)
    n3297 = xnode "Read/Write Control"("FPGA VI Reference In"=w4401) -> ("FPGA VI Reference Out"=w4400:T31, "BD1 Frequency Out 1"=w4399:u64)  [unwired: 1 in, 1 out]
    n3298 = local read "Data Period (s)"() -> (w4537:dbl)
    n3299 = local read "BD 1 Frequency 2 (MHz)"() -> (w4570:dbl)
    n3300 = local read "BD 1 Frequency 1 (MHz)"() -> (w4571:dbl)
    n3301 = Decimate 1D Array(w4578) -> (w4602:dbl[], w4601:dbl[], w4599:dbl[], w4598:dbl[])  [unwired: 9 out]
    n3302 = Multiply(x=w4537, y="Trap Pos. Disp. Downsample") -> (x*y=w4535:dbl)
    n3303 = Divide(x=w4602, y=w4601) -> (x/y=w4603:dbl[])
    n3304 = Divide(x=w4599, y=w4598) -> (x/y=w4600:dbl[])
    n3305 = local read "AOM X Cal (nm/MHz)"() -> (w4568:dbl)
    n3306 = Split 1D Array(array=w4603, index="N El. to Ave.") -> (second subarray=w4606:dbl[])  [unwired: 1 out]
    n3307 = Split 1D Array(array=w4600, index="N El. to Ave.") -> (second subarray=w4605:dbl[])  [unwired: 1 out]
    n3308 = Multiply(x=w4537, y="Trap Disp. Downsample") -> (x*y=w4616:dbl)
    "Display Period (s)" <- w4616
    n3309 = for "Trap AI" {
      tunnel: [w5430] -> w4446 mode=indexing
      tunnel: w4614 -> [w5421]
      tunnel: "Trap Disp. Downsample" -> [w5428]
      tunnel: w4673 -> [w5426] mode=indexing
      tunnel: w4537 -> [w5425]
      tunnel: w4672 -> [w5424] mode=indexing
      tunnel: [w5423] -> w4647 mode=indexing
      tunnel: w4616 -> [w5422]
      workers-P: _ -> [_]
      n3310 = Bundle By Name("Y"=w5426, "dt"=w5425) -> (w5427:waveform(dbl))  [unwired: 1 out]
      n3311 = Set Waveform Attribute(5:w5424, 6:"NI_ChannelName" ("name"), 7:w5427) -> (3:w5423:waveform(dbl))  [unwired: 1 in, 2 out]
      n3312 = call "downsample 1D array - double.vi"("Ave N"=w5428, "Array In"=w5426) -> ("Array Out"=w5429:dbl[])  [unwired: 1 out]
      n3313 = Bundle By Name(cluster=w5423, "t0"=w5421, "Y"=w5429, "dt"=w5422) -> (w5430:waveform(dbl))
    }
    n3314 = Bundle("BD 1 Frequency 1 (MHz)"=w4571, "BD 1 Frequency 2 (MHz)"=w4570) -> (w4572:T61)  [unwired: 1 out]
    n3315 = call-poly <vilib>:"Mean.vi"("X"=w4605) -> ("mean"=w4593:dbl)  [unwired: 1 out]
    n3316 = call-poly <vilib>:"Mean.vi"("X"=w4606) -> ("mean"=w4594:dbl)  [unwired: 1 out]
    n3317 = local read "BD 1 Frequency 2 (MHz)"() -> (w4411:dbl)
    n3318 = Reciprocal(x=w4616) -> (1/x=→"Trap Disp. Freq. (Hz)":dbl)
    n3319 = Cluster To Array(cluster=w4572) -> (array=w4569:dbl[])
    n3320 = To Double Precision Float(number=w4399) -> (double precision float=w4404:dbl)
    n3321 = Multiply(x=w4402, y=w4403) -> (x*y=w4405:dbl)
    n3322 = local read "Trap X AI1 (DMA)"() -> (w4604:T16)
    n3323 = Multiply(x=w4404, y=w4405) -> (x*y=w4406:dbl)
    n3324 = local read "Data points/scans (MCL)"() -> (w4725:dbl)
    n3325 = To Fixed-Point(number=w4593) -> (fixed-point=w4591:fxp<+/-,16,1>)  [unwired: 1 in]
    n3326 = To Fixed-Point(number=w4594) -> (fixed-point=w4592:fxp<+/-,16,1>)  [unwired: 1 in]
    n3327 = Scale By Power Of 2(n=-48, x=w4406) -> (x*2^n=w4408:dbl)
    n3328 = Bundle("Trap 1 Pos.", "Trap 2 Pos.") -> (w4613:cluster{string, string})  [unwired: 1 out]
    n3329 = Divide(x=w4408, y=1000000.0) -> (x/y=w4410:dbl)
    n3330 = Bundle By Name(cluster=w4604, "Set 1"=w4592, "Set 2"=w4591) -> (→"Trap X AI1 (DMA)":T16)
    n3331 = Cluster To Array(cluster=w4613) -> (array=w4610:string[])
    n3332 = Subtract(x=w4411, y=w4410) -> (x-y=w4393:dbl)
    "Current deltaF (MHz)" <- w4393
    n3333 = Unbundle(w4478) -> (w4479:void[])  [unwired: 2 out]
    n3334 = Select(t=-1.0, s="Negate Y Axis", f=1.0) -> (s? t:f=w4554:dbl)
    n3335 = for "Trap Position" {
      tunnel: w4618 -> [w5068] mode=indexing
      tunnel: "Trap Pos. Disp. Downsample" -> [w5067]
      tunnel: w4535 -> [w5065]
      tunnel: w4614 -> [w5064]
      tunnel: w4610 -> [w5062] mode=indexing
      tunnel: [w5061] -> w4525 mode=indexing
      tunnel: w4569 -> [w5059] mode=indexing
      tunnel: w4568 -> [w5057]
      tunnel: w4554 -> [w5056]
      n3336 = call "downsample 1D array - double.vi"("Ave N"=w5067, "Array In"=w5068) -> ("Array Out"=w5066:dbl[])  [unwired: 1 out]
      n3337 = Subtract(x=w5066, y=w5059) -> (x-y=w5060:dbl[])
      n3338 = Multiply(x=w5057, y=w5060) -> (x*y=w5058:dbl[])
      n3339 = Multiply(x=w5056, y=w5058) -> (x*y=w5055:dbl[])
      n3340 = Bundle By Name("Y"=w5055, "dt"=w5065, "t0"=w5064) -> (w5063:waveform(dbl))  [unwired: 1 out]
      n3341 = Set Waveform Attribute(5:w5062, 6:"NI_ChannelName" ("name"), 7:w5063) -> (3:w5061:waveform(dbl))  [unwired: 1 in, 2 out]
    }
    n3342 = To Double Precision Float(number=w4479) -> (double precision float=w4670:dbl[])
    n3343 = local read "Display Period (s)"() -> (w4662:dbl)
    n3344 = Increment(x=w4725) -> (x+1=w4726:dbl)
    n3345 = Index Array(array=w4525, index=0) -> (element=w4529:waveform(dbl))
    n3346 = Index Array(array=w4525, index=1) -> (element=w4524:waveform(dbl))
    n3347 = feedback #10(w4726) -> (w4729:dbl)
    n3348 = Select(t=0, s=w4716, f=w4729) -> (s? t:f=w4722:dbl)
    n3349 = Array Size(array=w4670) -> (size(s)=w4728:i32)
    n3350 = Add(x=w4728, y=w4722) -> (x+y=w4723:dbl)
    n3351 = Unbundle By Name(w4529) -> ("Y"=w4530:dbl[])
    n3352 = Divide(x="Bead Sep. Int. Time (s)", y=w4662) -> (x/y=w4564:dbl)
    n3353 = Add(x=w4530, y="FB Trap Pos Offset") -> (x+y=w4528:dbl[])
    "T1 x pos data" <- w4528
    n3354 = Greater?(x=w4723, y=w4725) -> (0:w4724:bool)
    n3355 = feedback #11(w4528) -> (w4566:dbl[])
    n3356 = Build Array (concatenate)(w4528, w4566) -> (w4565:dbl[])
    n3357 = Bundle By Name(cluster=w4529, "Y"=w4528) -> (w4527:waveform(dbl))
    n3358 = Select(t=w4722, s=w4724, f=w4723) -> (s? t:f=w4721:dbl)
    n3359 = feedback-in #10(w4721) -> ()
    n3360 = local read "MCL Scanning"() -> (w4719:bool)
    n3361 = Bundle(w4527, w4524) -> (w4523:cluster{waveform(dbl), waveform(dbl)})  [unwired: 1 out]
    n3362 = Index Array(array=w4446, index="index 1") -> (element=w4468:waveform(dbl))
    n3363 = Index Array(array=w4446, index="index 2") -> (element=w4472:waveform(dbl))
    n3364 = Split 1D Array(array=w4565, index=w4564) -> (first subarray=w4558:dbl[])  [unwired: 1 out]
    n3365 = feedback-in #11(w4558) -> ()
    n3366 = Unbundle By Name(w4468) -> ("Y"=w4467:dbl[])
    n3367 = Unbundle By Name(w4472) -> ("Y"=w4471:dbl[])
    n3368 = Not(x=w4724) -> (.not. x?=w4718:bool)
    n3369 = Cluster To Array(cluster=w4523) -> (array=w4503:waveform(dbl)[])
    "Trap Positions" <- w4503
    n3370 = call-poly <vilib>:"Mean.vi"("X"=w4558) -> ("mean"=w4557:dbl)  [unwired: 1 out]
    "Mean T1 Position (nm)" <- w4557
    n3371 = Subtract(x=w4558, y=w4557) -> (x-y=w4563:dbl[])
    n3372 = Square(x=w4563) -> (x^2=w4562:dbl[])
    n3373 = And(x=w4718, y=w4719) -> (x .and. y?=w4720:bool)
    n3374 = call-poly <vilib>:"Mean.vi"("X"=w4562) -> ("mean"=w4561:dbl)  [unwired: 1 out]
    n3375 = call-poly <vilib>:"Mean.vi"("X"=w4467) -> ("mean"=→"Trap 1 sum mean":dbl)  [unwired: 1 out]
    n3376 = call-poly <vilib>:"Mean.vi"("X"=w4471) -> ("mean"=→"Trap 2 sum mean":dbl)  [unwired: 1 out]
    n3377 = Square Root(x=w4561) -> (sqrt(x)=w4560:dbl)
    n3378 = Or(x=w4720, y=w4716) -> (x .or. y?=w4717:bool)
    n3379 = Build Array (concatenate)(w4645, w4446) -> (w4426:waveform(dbl)[])
    "All Signals" <- w4426
    n3380 = Equal?(x="Tab Control 6", y=T51."High Res Display") -> (x = y?=w4674:bool)
    n3381 = case shown="False" "X or Y?" {
      tunnel: w4446 -> [w4887 w4893]
      tunnel: [w4888 w4892] -> w4441
      tunnel: [w4886 w4891] -> w4438
      frame False {
        n3382 = Index Array(array=w4887, index=0) -> (element=w4888:waveform(dbl))
        n3383 = Index Array(array=w4887, index=3) -> (element=w4886:waveform(dbl))
      }
      frame True {
        n3384 = Index Array(array=w4893, index=1) -> (element=w4892:waveform(dbl))
        n3385 = Index Array(array=w4893, index=4) -> (element=w4891:waveform(dbl))
      }
    }
    n3386 = Multiply(x=10.0, y=w4560) -> (x*y=→"Trap 1 Position RMS (A)":dbl)
    n3387 = case "For displaying the high resolution display (no downsampling)" shown="True" w4674 {
      tunnel: w4647 -> [_ w5088]
      frame False {
      }
      frame True {
        n3388 = Index Array(array=w5088, index="High Res. Display") -> (element=w5089:waveform(dbl))
        n3389 = call <vilib>:"Std Deviation and Variance.vi"("X"=w5089) -> ("mean"=w5096:dbl, "standard deviation"=w5101:dbl)  [unwired: 1 in, 1 out]
        "Mean Intensity" <- w5096
        "Sigma" <- w5101
        n3390 = Subtract(x=w5089, y=w5096) -> (x-y=w5095:waveform(dbl))
        n3391 = Select(t=w5095, s="Subtract mean", f=w5089) -> (s? t:f=→"1 Channel":waveform(dbl))
        n3392 = Divide(x=w5101, y=w5096) -> (x/y=→"Sigma/Mean":dbl)
        n3393 = feedback #12(1) -> (w5090:i32)
        n3394 = Greater Or Equal?(x=w5090, y="Slow mean N ave.") -> (x >= y?=w5103:bool)
        n3395 = Increment(x=w5090) -> (x+1=w5105:i32)
        n3396 = Select(t=1, s=w5103, f=w5105) -> (s? t:f=w5092:i32)
        n3397 = feedback-in #12(w5092) -> ()
        n3398 = feedback #13() -> (w5093:waveform(dbl))  [unwired: 1 out]
        n3399 = case shown="Default" w5090 {
          tunnel: [w5108 w5111] -> w5094
          tunnel: w5093 -> [w5110 _]
          tunnel: w5089 -> [w5109 w5111]
          frame Default {
            n3400 = call-poly <vilib>:"Append Waveforms.vi"("waveform B"=w5109, "waveform A"=w5110) -> ("waveform out"=w5108:waveform(dbl))  [unwired: 1 in, 8 out]
          }
          frame 1 {
          }
        }
        n3401 = feedback-in #13(w5094) -> ()
        n3402 = case shown="True" w5103 {
          tunnel: w5094 -> [_ w5107]
          frame False {
          }
          frame True {
            n3403 = call-poly <vilib>:"Mean.vi"("X"=w5107) -> ("mean"=→"Slow mean":dbl)  [unwired: 1 out]
          }
        }
      }
    }
    n3404 = case "For plotting results of scanning MCL (fluorescence and detection laser images)" shown="True" w4717 {
      tunnel: w4716 -> [_ w5203]
      tunnel: w4725 -> [_ _]
      tunnel: w4647 -> [_ w5299]
      tunnel: w4627 -> [_ w5231]
      tunnel: w4478 -> [_ w5209]
      frame False {
      }
      frame True {
        w5169 = u32 0 items=["Horizontal", "Vertical", "Central", "1st Diagonal", "2nd Diagonal"] ("Type of Symmetry")
        w5176 = u32 0 items=["Horizontal", "Vertical", "Central", "1st Diagonal", "2nd Diagonal"] ("Type of Symmetry")
        w5183 = u32 0 items=["Horizontal", "Vertical", "Central", "1st Diagonal", "2nd Diagonal"] ("Type of Symmetry")
        w5186 = u32 0 items=["Horizontal", "Vertical", "Central", "1st Diagonal", "2nd Diagonal"] ("Type of Symmetry")
        w5193 = u32 0 items=["Horizontal", "Vertical", "Central", "1st Diagonal", "2nd Diagonal"] ("Type of Symmetry")
        n3405 = Unbundle(w5209) -> (w5208:void[], w5206:void[], w5204:u32)
        n3406 = To Double Precision Float(number=w5208) -> (double precision float=w5207:dbl[])
        n3407 = To Double Precision Float(number=w5206) -> (double precision float=w5205:dbl[])
        n3408 = To Double Precision Float(number=w5204) -> (double precision float=w5197:dbl)
        n3409 = Index Array(array=w5299, index=10) -> (element=w5305:waveform(dbl))
        n3410 = Index Array(array=w5299, index=11) -> (element=w5302:waveform(dbl))
        n3411 = local read "Cycles/step (MCL)"() -> (w5261:u64)
        n3412 = Index Array(array=w5299, index="Channel") -> (element=w5301:waveform(dbl))
        n3413 = Unbundle(w5231) -> ("New Image"=w5230:T2, "New Image"=w5229:T2, "New Image"=w5210:T2, "New Image"=w5211:T2, "New Image"=w5212:T2)
        n3414 = local read "Scan steps (MCL)"() -> (w5199:u64)
        n3415 = Unbundle By Name(w5305) -> ("Y"=w5263:dbl[])
        n3416 = Unbundle By Name(w5302) -> ("Y"=w5265:dbl[])
        n3417 = local read "Scan lines (y)"() -> (w5200:u64)
        n3418 = local read "N APD Samp/step"() -> (w5202:dbl)
        n3419 = Unbundle By Name(w5301) -> ("Y"=w5270:dbl[])
        n3420 = call "downsample 1D array - double.vi"("Ave N"=w5261, "Array In"=w5263) -> ("Array Out"=w5262:dbl[])  [unwired: 1 out]
        n3421 = call "downsample 1D array - double.vi"("Ave N"=w5261, "Array In"=w5265) -> ("Array Out"=w5264:dbl[])  [unwired: 1 out]
        n3422 = call "downsample 1D array - double.vi"("Ave N"=w5261, "Array In"=w5270) -> ("Array Out"=w5269:dbl[])  [unwired: 1 out]
        n3423 = Multiply(x=w5199, y=u64 2) -> (x*y=w5201:u64)
        n3424 = feedback #14(w5205) -> (w5249:dbl[])
        n3425 = Build Array (concatenate)(w5249, w5205) -> (w5248:dbl[])
        n3426 = feedback #15(w5197) -> (w5198:dbl)
        n3427 = Build Array(w5198, w5197) -> (w5196:dbl[])
        n3428 = Select(t=w5205, s=w5203, f=w5248) -> (s? t:f=w5233:dbl[])
        n3429 = feedback-in #14(w5233) -> ()
        n3430 = Select(t=w5197, s=w5203, f=w5196) -> (s? t:f=w5214:dbl)
        n3431 = feedback-in #15(w5214) -> ()
        n3432 = feedback #16(w5207) -> (w5324:dbl[])
        n3433 = Build Array (concatenate)(w5324, w5207) -> (w5307:dbl[])
        n3434 = Select(t=w5207, s=w5203, f=w5307) -> (s? t:f=w5311:dbl[])
        n3435 = feedback-in #16(w5311) -> ()
        n3436 = feedback #17(w5262) -> (w5313:dbl[])
        n3437 = Build Array (concatenate)(w5313, w5262) -> (w5304:dbl[])
        n3438 = feedback #18(w5269) -> (w5322:dbl[])
        n3439 = Build Array (concatenate)(w5322, w5269) -> (w5321:dbl[])
        n3440 = feedback #19(w5264) -> (w5315:dbl[])
        n3441 = Build Array (concatenate)(w5315, w5264) -> (w5316:dbl[])
        n3442 = Select(t=w5262, s=w5203, f=w5304) -> (s? t:f=w5266:dbl[])
        n3443 = feedback-in #17(w5266) -> ()
        n3444 = Select(t=w5269, s=w5203, f=w5321) -> (s? t:f=w5268:dbl[])
        n3445 = feedback-in #18(w5268) -> ()
        n3446 = Select(t=w5264, s=w5203, f=w5316) -> (s? t:f=w5267:dbl[])
        n3447 = feedback-in #19(w5267) -> ()
        n3448 = call "integrate 1D array interval - double.vi"("Ave N"=w5202, "Array In"=w5233) -> ("Array Out"=w5244:dbl[])  [unwired: 1 out]
        n3449 = call "integrate 1D array interval - double.vi"("Ave N"=w5202, "Array In"=w5214) -> ("Array Out"=w5225:dbl[])  [unwired: 1 out]
        n3450 = call "integrate 1D array interval - double.vi"("Ave N"=w5202, "Array In"=w5311) -> ("Array Out"=w5310:dbl[])  [unwired: 1 out]
        n3451 = Array Size(array=w5244) -> (size(s)=w5245:i32)
        n3452 = Array Size(array=w5225) -> (size(s)=w5226:i32)
        n3453 = Array Size(array=w5310) -> (size(s)=w5312:i32)
        n3454 = Multiply(x=w5200, y=w5201) -> (x*y=w5247:u64)
        n3455 = Multiply(x=w5200, y=w5201) -> (x*y=w5228:u64)
        n3456 = Multiply(x=w5200, y=w5201) -> (x*y=w5320:u64)
        n3457 = Subtract(x=w5247, y=w5245) -> (x-y=w5238:u64)
        n3458 = call-poly <vilib>:"Mean.vi"("X"=w5244) -> ("mean"=w5235:dbl)  [unwired: 1 out]
        n3459 = Subtract(x=w5228, y=w5226) -> (x-y=w5219:u64)
        n3460 = call-poly <vilib>:"Mean.vi"("X"=w5225) -> ("mean"=w5216:dbl)  [unwired: 1 out]
        n3461 = Subtract(x=w5320, y=w5312) -> (x-y=w5260:u64)
